vi "Gen Stage 1 Update Name.vi"(4 "Documentation":T1, 6 "Channels to Create":T2[](array[typedef]), 7 "Staus":refnum<vi>, 8 "error in":errorcluster, 9 "Overlay Icon":refnum<class "Icon.lvclass">, 10 "New Subname":string, 11 "Template Project Path":path) -> (0 "error out":errorcluster)   [LabVIEW 2021, in "Plugin Generator.lvlib"]
uses:
  Plugin Generator.lvlib
  <vilib>/CIF Foundation/CIF Core/Channels/ChannelRegistrar/typedef/Channel Definition for Scripting.ctl
  <vilib>/CIF Foundation/CIF Channels Core/CIFChannels/Typedef/Direction.ctl
  <vilib>/CIF Foundation/CIF Core/Channels/ChannelRegistrar/typedef/Registered Channel Types.ctl
  <vilib>/LabVIEW Icon API/lv_icon/Classes/Icon/Icon.lvclass
  Typedef/Documentation Info.ctl
  <vilib>/CIF Foundation/CIF LabVIEW Scripting/LV Scripting/LV Scripting Utilities.lvlib
  <vilib>/CIF Foundation/CIF Channels Core/CIFChannels/CIFChannels.lvclass
  <vilib>/CIF Foundation/CIF Core/Channels/ChannelRegistrar/ChannelRegistrar.lvlib
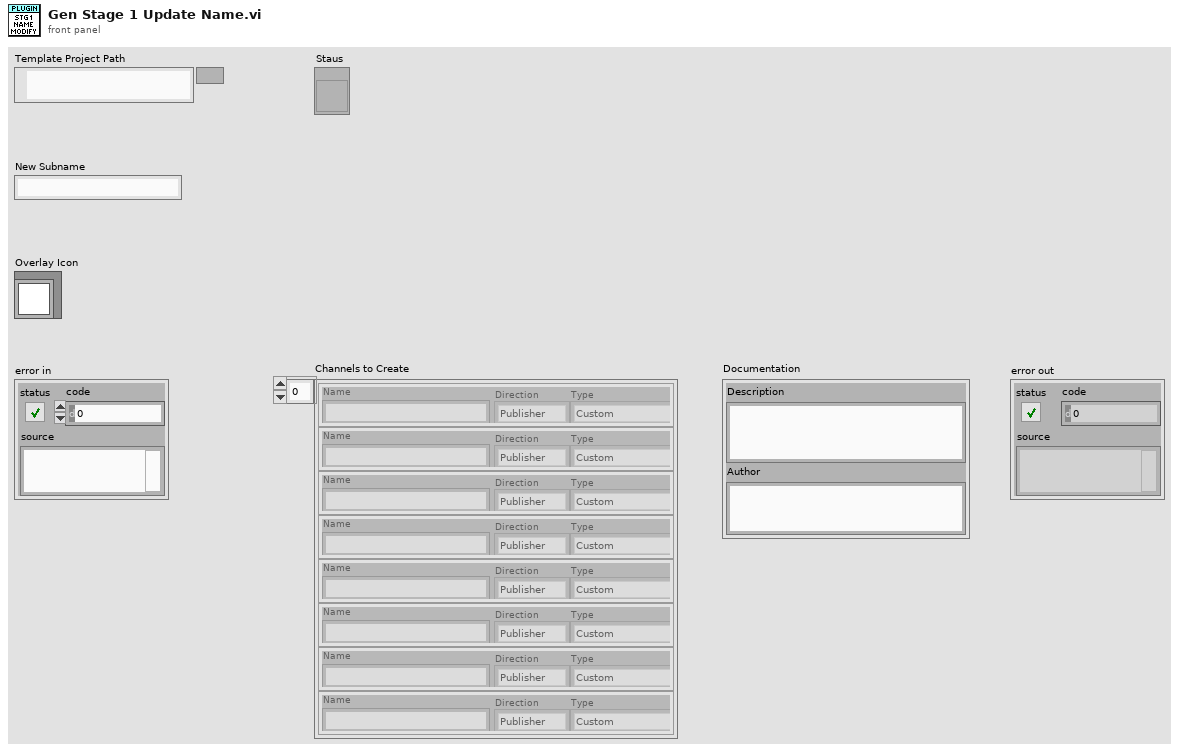
[diagram p1: front panel]
types:
  T1 = typedef "Plugin Generator.lvlib/Documentation Info.ctl" = cluster{"Description":string, "Author":string}
  T2 = typedef "ChannelRegistrar.lvlib/Channel Definition for Scripting.ctl" = cluster{"Name":string, "Direction":T3, "Type":T4}
  T3 = typedef "CIFChannels.lvclass/Direction.ctl" = enum16{"Publisher", "Subscriber"}
  T4 = typedef "ChannelRegistrar.lvlib/Registered Channel Types.ctl" = enum16{"Custom", "Double_Tag", "I64_Tag", "U64_Tag", "U8_FIFO", "CAN_FIFO", "L2Enet_FIFO", "DAQ_FIFO", "Universal_FIFO", "String_Tag"}
  T5 = cluster{"Library Name":string, "Update Folder Name":bool}[]
  T6 = typedef "LV Scripting Utilities.lvlib/Target References.ctl" = cluster{"Target Reference":refnum<vi>, "VI References":refnum<vi>[], "Library References":refnum<vi>[], "Build References":refnum<vi>[]}
  T7 = typedef "LV Scripting Utilities.lvlib/Library Map.ctl" = map{string, refnum<vi>}
  T8 = typedef "LV Scripting Utilities.lvlib/VI Map.ctl" = map{string, refnum<vi>}
  T9 = typedef "Plugin Generator.lvlib/Proto Names.ctl" = cluster{"PascalCase":string, "snake_case":string}
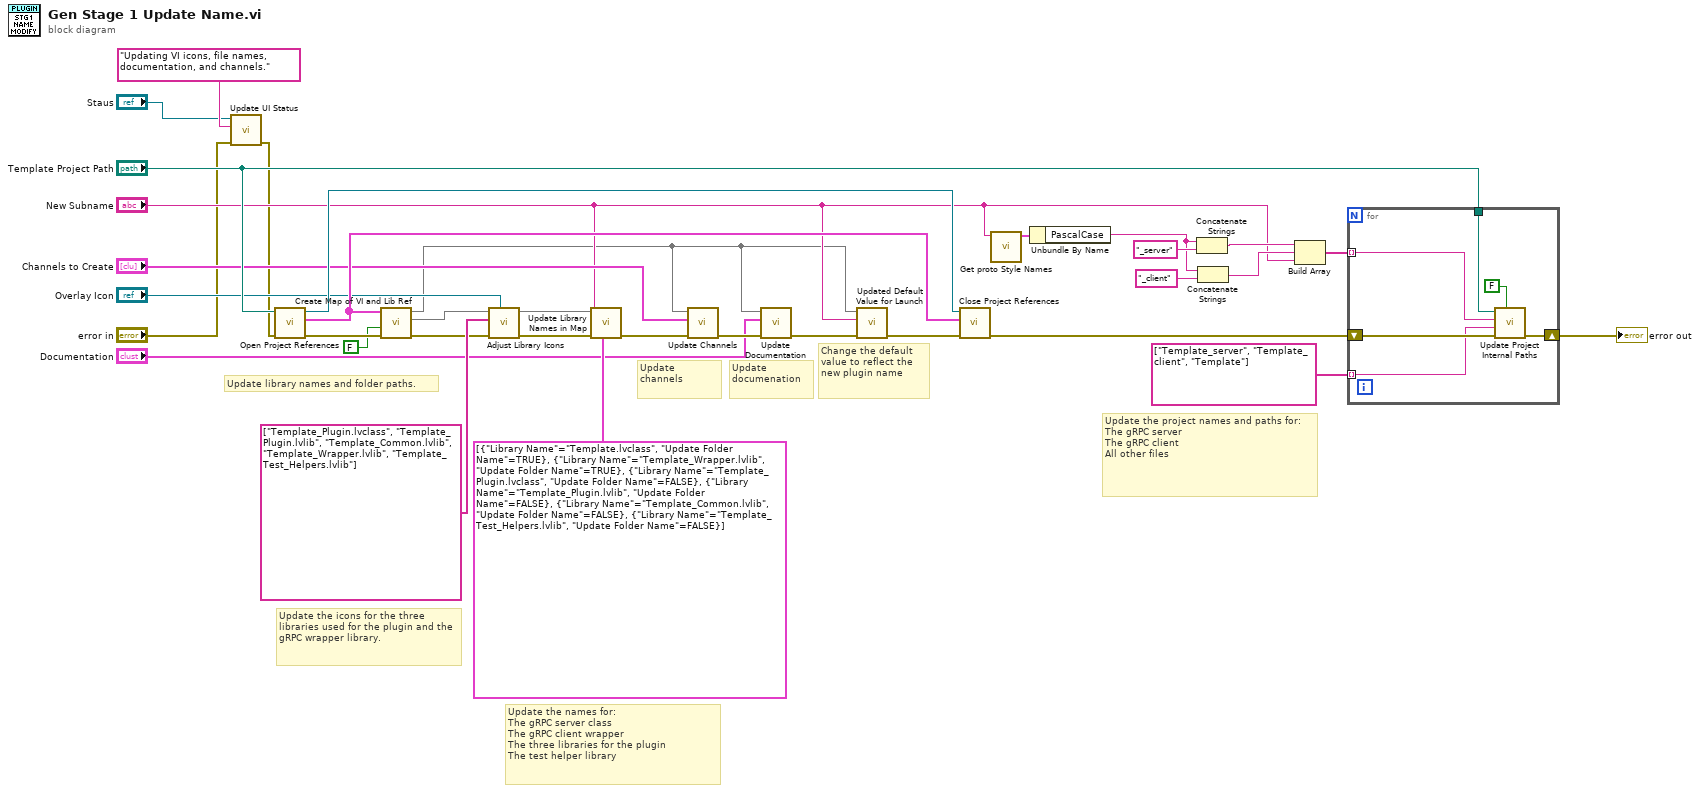
[diagram p0: block diagram]
diagram:
  # "Update documenation"
  # "Update the project names and paths for:\nThe gRPC server \nThe gRPC client \nAll other files"
  # "Update channels"
  # "Update library names and folder paths."
  # "Change the default value to reflect the new plugin name"
  # "Update the names for:\nThe gRPC server class\nThe gRPC client wrapper\nThe three libraries for the plugin\nThe test helper library"
  # "Update the icons for the three libraries used for the plugin and the gRPC wrapper library."
  n1 = call "Update UI Status.vi"("error in"="error in", "Status to Display"="Updating VI icons, file names, documentation, and channels." ("To display"), "String in"="Staus") -> ("error out"=w8:errorcluster)  [unwired: 8 in]
  n2 = call <vilib>:"Open Project References.vi"("error in"=w8, "Project Path"="Template Project Path") -> ("error out"=w27:errorcluster, "VI, Library, and Build References"=w24:T6[], "Project Reference"=w25:refnum<vi>)  [unwired: 7 in]
  n3 = call <vilib>:"Create Map of VI and Lib Ref.vi"("error in"=w27, "RT Target"=FALSE, "VI, Library, and Build References"=w24) -> ("error out"=w31:errorcluster, "Library Map"=w32:T7, "VI Map"=w2:T8)  [unwired: 5 in, 1 out]
  n4 = call <vilib>:"Adjust Library Icons.vi"("Overlay Icon"="Overlay Icon", "error in"=w31, "Library Names"=string[] ["Template_Plugin.lvclass", "Template_Plugin.lvlib", "Template_Common.lvlib", "Template_Wrapper.lvlib", "Template_Test_Helpers.lvlib"], "Library Map in"=w32) -> ("error out"=w5:errorcluster, "Library Map out"=w30:map{string, refnum<vi>})  [unwired: 5 in, 1 out]
  n5 = call <vilib>:"Update Library Names in Map.vi"("Libraries"=T5 [{"Library Name"="Template.lvclass", "Update Folder Name"=TRUE}, {"Library Name"="Template_Wrapper.lvlib", "Update Folder Name"=TRUE}, {"Library Name"="Template_Plugin.lvclass", "Update Folder Name"=FALSE}, {"Library Name"="Template_Plugin.lvlib", "Update Folder Name"=FALSE}, {"Library Name"="Template_Common.lvlib", "Update Folder Name"=FALSE}, {"Library Name"="Template_Test_Helpers.lvlib", "Update Folder Name"=FALSE}], "error in"=w5, "New Subname"="New Subname", "Library Map"=w30) -> ("error out"=w22:errorcluster)  [unwired: 6 in, 1 out]
  n6 = call "Update Channels.vi"("error in"=w22, "Channels to Create"="Channels to Create", "VI Map"=w2) -> ("error out"=w4:errorcluster)  [unwired: 8 in]
  n7 = call "Update Documentation.vi"("error in"=w4, "Documentation"="Documentation", "VI Map"=w2) -> ("error out"=w3:errorcluster)  [unwired: 8 in]
  n8 = call "Updated Default Value for Launch.vi"("error in"=w3, "New Subname"="New Subname", "Name to VI Map"=w2) -> ("error out"=w26:errorcluster)  [unwired: 8 in]
  n9 = call <vilib>:"Close Project References.vi"("error in"=w26, "VI, Library, and Build References"=w24, "Project Reference"=w25) -> ("error out"=w19:errorcluster)  [unwired: 8 in]
  n10 = call "Get proto Style Names.vi"("Input Name"="New Subname") -> ("Proto Names"=w18:T9)  [unwired: 10 in]
  n11 = Unbundle By Name(w18) -> ("PascalCase"=w16:string)
  n12 = Concatenate Strings(w16, "_server" ("Replace Subname")) -> (w14:string)
  n13 = Concatenate Strings(w16, "_client" ("Replace Subname")) -> (w13:string)
  n14 = Build Array(w14, w13, "New Subname") -> (w12:string[])
  n15 = for {
    tunnel: "Template Project Path" -> [w39]
    shift-right: [w40] -> w34
    shift-left: w19 -> [w37]
    tunnel: w12 -> [w35] mode=indexing
    tunnel: string[] ["Template_server", "Template_client", "Template"] -> [w36] mode=indexing
    n16 = call <vilib>:"Update Project Internal Paths.vi"("Rename Project"=FALSE, "error in (no error)"=w37, "Replace Subname"=w36, "New Subname"=w35, "Project Path"=w39) -> ("error out"=w40:errorcluster)  [unwired: 6 in]
  }
  "error out" <- w34
